vi "Update Trig Line.vi"(8 "error in (no error)":errorcluster, 9 "PB Trigger Line":i32, 10 "Triggering":bool[](array[boolean]), 11 "Master Device in":refnum<class "Master Device.lvclass">) -> (0 "error out":errorcluster, 3 "Master Device out":refnum<class "Master Device.lvclass">)   [LabVIEW 2013, in "Master Device.lvclass"]
uses:
  Master Device.lvclass
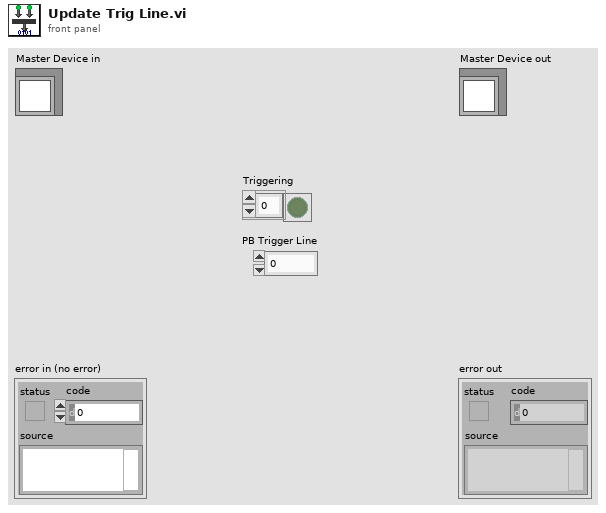
[diagram p1: front panel]
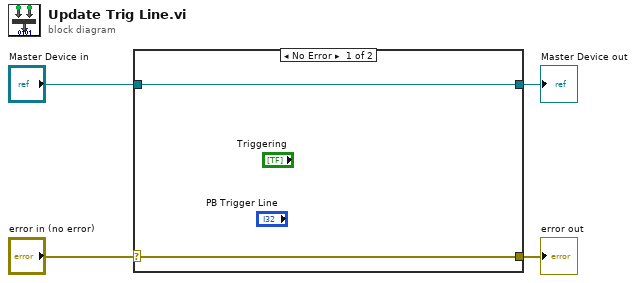
[diagram p0: block diagram]
diagram:
  n1 = case shown="No Error" "error in (no error)" {
    selector: "error in (no error)" -> [w6 w7]
    tunnel: [w6 w7] -> w3
    tunnel: [w5 w8] -> w1
    tunnel: "Master Device in" -> [w5 w8]
    frame No Error {
    }
    frame Error {
    }
  }
  "error out" <- w3
  "Master Device out" <- w1
